vi "Tool Objects.vi"(8 "error in (no error)":errorcluster, 11 "Tool Data in":refnum<class "Tool Data.lvclass">) -> (0 "error out":errorcluster, 3 "Tool Data out":refnum<class "Tool Data.lvclass">)   [LabVIEW 2019, in "Tool Data.lvclass"]
uses:
  Tool Data.lvclass
  Tool Data.lvclass/Tool Data.ctl
  Tool Path/Tool Path.lvclass
  Tool Funnel/Tool Funnel.lvclass
  Tool Rectangle/Tool Rectangle.lvclass
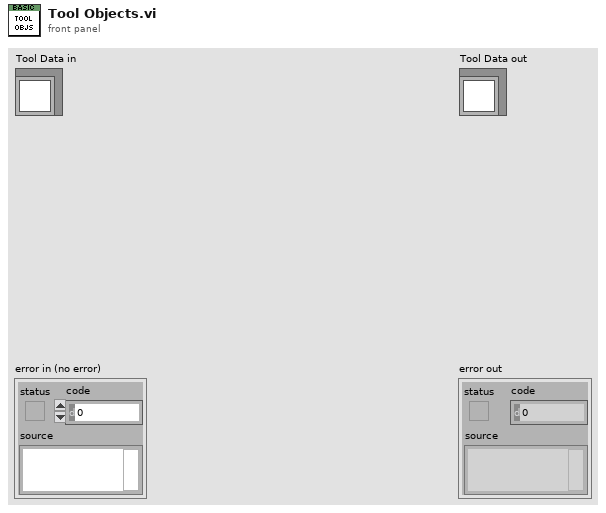
[diagram p1: front panel]
types:
  T1 = typedef "Setting Database.lvclass/PublicEvents--Setting Database.RectanglesUpdated.ctl" = refnum<class "Rectangle Settings.lvclass">[]
  T2 = typedef "Setting Database.lvclass/PublicEvents--Setting Database.FunnelsUpdated.ctl" = refnum<class "Funnel Settings.lvclass">[]
  T3 = typedef "Setting Database.lvclass/PublicEvents--Setting Database.PathsUpdated.ctl" = refnum<class "Path Settings.lvclass">[]
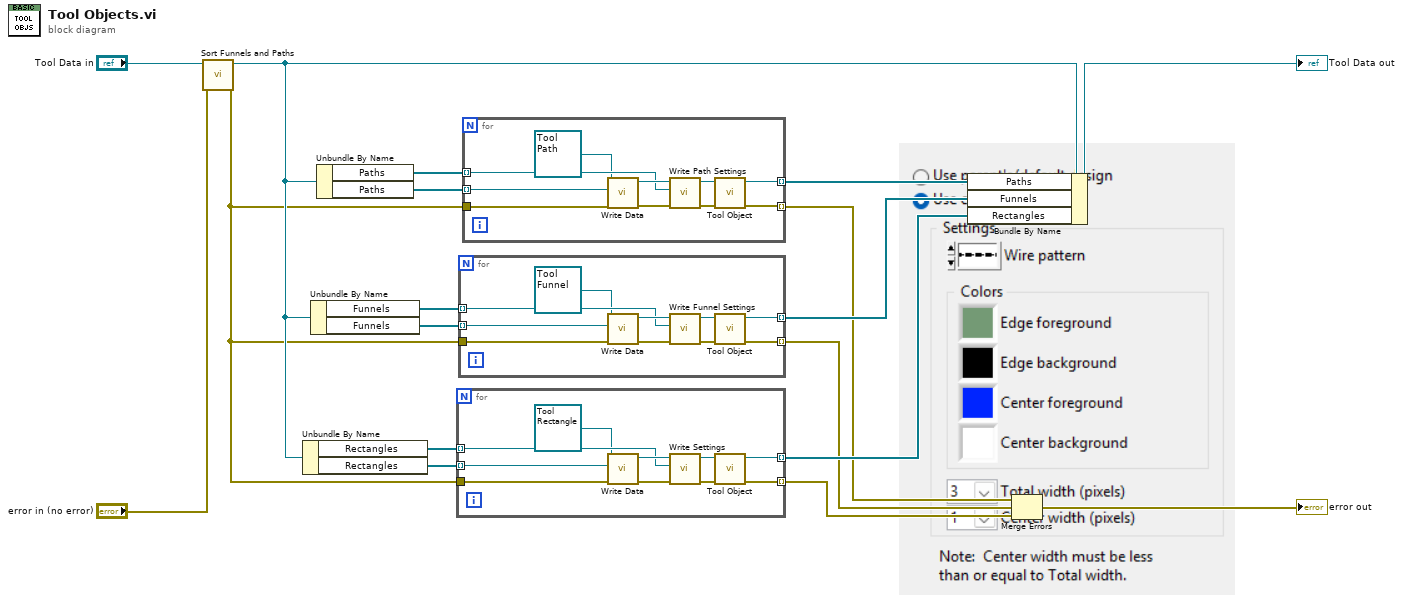
[diagram p0: block diagram]
diagram:
  n1 = call "Sort Funnels and Paths.vi"("error in (no error)"="error in (no error)", "Tool Data in"="Tool Data in") -> ("error out"=w2:errorcluster, "Tool Data out"=w10:refnum<class "Tool Data.lvclass">)  [unwired: 8 in]
  n2 = Unbundle By Name(w10) -> ("Rectangles"=w12:T1, "Rectangles"=w11:refnum<class "Rectangle.lvclass">[])
  n3 = Unbundle By Name(w10) -> ("Funnels"=w13:T2, "Funnels"=w14:refnum<class "Path.lvclass">[])
  n4 = Unbundle By Name(w10) -> ("Paths"=w16:T3, "Paths"=w15:refnum<class "Path.lvclass">[])
  n5 = for {
    tunnel: w12 -> [w22] mode=indexing
    tunnel: w11 -> [w23] mode=indexing
    tunnel: [w21] -> w6 mode=indexing
    tunnel: w2 -> [w20]
    tunnel: [w28] -> w3 mode=indexing
    n6 = call-dynamic "Write Data.vi"("error in (no error)"=w20, "Rectangle.lvclass"=w23, "Tool Rectangle in"=refnum<class "Tool Rectangle.lvclass"> refnum) -> ("error out"=w26:errorcluster, "Tool Rectangle out"=w27:refnum<class "Tool Rectangle.lvclass">)  [unwired: 7 in]
    n7 = call-dynamic "Write Settings.vi"("error in (no error)"=w26, "Rectangle Settings.lvclass"=w22, "Tool Rectangle in"=w27) -> ("error out"=w24:errorcluster, "Tool Rectangle out"=w25:refnum<class "Tool Rectangle.lvclass">)  [unwired: 7 in]
    n8 = call-dynamic "Tool Object.vi"("error in (no error)"=w24, "Tool Rectangle in"=w25) -> ("error out"=w28:errorcluster, "Tool Rectangle out"=w21:refnum<class "Tool Rectangle.lvclass">)  [unwired: 8 in]
  }
  n9 = for {
    tunnel: w13 -> [w32] mode=indexing
    tunnel: w14 -> [w33] mode=indexing
    tunnel: [w30] -> w7 mode=indexing
    tunnel: w2 -> [w35]
    tunnel: [w31] -> w4 mode=indexing
    n10 = call-dynamic "Write Data.vi"("error in (no error)"=w35, "Path.lvclass"=w33, "Tool Path in"=refnum<class "Tool Funnel.lvclass"> refnum ("Tool Funnel in")) -> ("error out"=w38:errorcluster, "Tool Path out"=w34:refnum<class "Tool Funnel.lvclass">)  [unwired: 7 in]
    n11 = call-dynamic "Write Funnel Settings.vi"("error in (no error)"=w38, "Funnel Settings.lvclass"=w32, "Tool Funnel in"=w34) -> ("error out"=w36:errorcluster, "Tool Funnel out"=w37:refnum<class "Tool Funnel.lvclass">)  [unwired: 7 in]
    n12 = call-dynamic "Tool Object.vi"("error in (no error)"=w36, "Tool Funnel in"=w37) -> ("error out"=w31:errorcluster, "Tool Funnel out"=w30:refnum<class "Tool Funnel.lvclass">)  [unwired: 8 in]
  }
  n13 = for {
    tunnel: w16 -> [w43] mode=indexing
    tunnel: w15 -> [w44] mode=indexing
    tunnel: [w40] -> w8 mode=indexing
    tunnel: w2 -> [w45]
    tunnel: [w41] -> w5 mode=indexing
    n14 = call-dynamic "Write Data.vi"("error in (no error)"=w45, "Path.lvclass"=w44, "Tool Path in"=refnum<class "Tool Path.lvclass"> refnum) -> ("error out"=w47:errorcluster, "Tool Path out"=w48:refnum<class "Tool Path.lvclass">)  [unwired: 7 in]
    n15 = call-dynamic "Write Path Settings.vi"("error in (no error)"=w47, "Path Settings.lvclass"=w43, "Tool Path in"=w48) -> ("error out"=w42:errorcluster, "Tool Path out"=w46:refnum<class "Tool Path.lvclass">)  [unwired: 7 in]
    n16 = call-dynamic "Tool Object.vi"("error in (no error)"=w42, "Tool Path in"=w46) -> ("error out"=w41:errorcluster, "Tool Path out"=w40:refnum<class "Tool Path.lvclass">)  [unwired: 8 in]
  }
  n17 = Bundle By Name(cluster=w10, "Paths"=w8, "Funnels"=w7, "Rectangles"=w6) -> (→"Tool Data out":refnum<class "Tool Data.lvclass">)
  n18 = Merge Errors(w5, w4, w3) -> (→"error out":errorcluster)
